vi "wd_append (Time).vi"(6 "data type":T7, 7 "data":timestamp[](array[timestamp]), 8 "error in (no error)":errorcluster, 9 "channel index":u32, 11 "meta in":T1={"TargetFile"=path "", "StreamMode"=enum."File", "Append?"=FALSE, "ChunkSize"=0, "TimeColumnMode"=enum."Empty", "TimestampFormat"="", "AbsoluteTime?"=FALSE, "FileAttribute "={"Creator"="", "Title"="", "SheetName"=""}, "Column"=[], "FileRef"=refnum, "MemoryRef"=[], "RecordInfo"=[], " ChannelPreviousInfo"=[], "ChannelFirstRecord"=[], "PredefinedFormattedValueLength"=20, "DiskTemplate"={"XMLRef"=[refnum, refnum, refnum, refnum, refnum, refnum], "ZipPath"=path "", "MetaFile"={"Ref"=refnum, "NextRow"=0, "NextPosition"=0, "Block"=[]}, "TempFolder"=path ""}}) -> (0 "error out":errorcluster, 3 "meta out":T1={"TargetFile"=path "", "StreamMode"=enum."File", "Append?"=FALSE, "ChunkSize"=0, "TimeColumnMode"=enum."Empty", "TimestampFormat"="", "AbsoluteTime?"=FALSE, "FileAttribute "={"Creator"="", "Title"="", "SheetName"=""}, "Column"=[], "FileRef"=refnum, "MemoryRef"=[], "RecordInfo"=[], " ChannelPreviousInfo"=[], "ChannelFirstRecord"=[], "PredefinedFormattedValueLength"=20, "DiskTemplate"={"XMLRef"=[refnum, refnum, refnum, refnum, refnum, refnum], "ZipPath"=path "", "MetaFile"={"Ref"=refnum, "NextRow"=0, "NextPosition"=0, "Block"=[]}, "TempFolder"=path ""}})   [LabVIEW 2017, in "NI_ExcelFile.lvlib"]
uses:
  <vilib>/express/express shared/NI_ExcelFile/NI_ExcelFile.lvlib
  <vilib>/express/express shared/NI_ExcelFile/Ctrls/DataType.ctl
  <vilib>/express/express shared/NI_ExcelFile/Ctrls/MainData.ctl
  <vilib>/express/express shared/NI_ExcelFile/Ctrls/StreamMode.ctl
  <vilib>/express/express shared/NI_ExcelFile/Ctrls/TimeColumnMode.ctl
  <vilib>/express/express shared/NI_ExcelFile/Ctrls/FileAttribute.ctl
  <vilib>/express/express shared/NI_ExcelFile/Ctrls/Columns.ctl
  <vilib>/express/express shared/NI_ExcelFile/Ctrls/ColumnInfo.ctl
  <vilib>/express/express shared/NI_ExcelFile/Ctrls/wd_recordInfo.ctl
  <vilib>/express/express shared/NI_ExcelFile/Ctrls/disk_TemplateFile.ctl
  <vilib>/express/express shared/NI_ExcelFile/Ctrls/meta_file.ctl
  <vilib>/express/express shared/NI_ExcelFile/Ctrls/meta_Block.ctl
  <vilib>/express/express shared/NI_ExcelFile/Ctrls/meta_BlockType.ctl
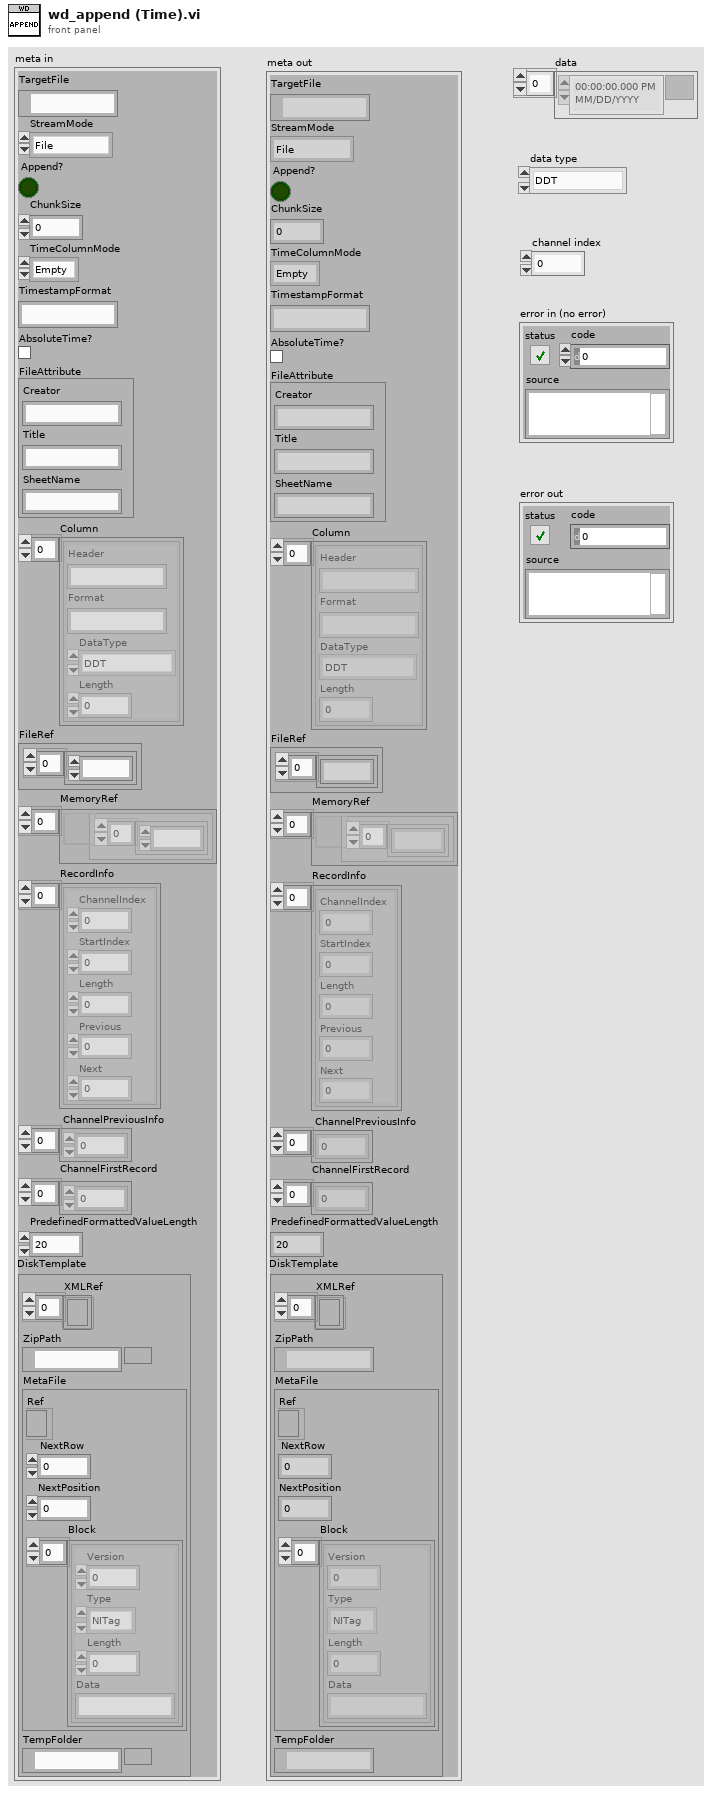
[diagram p1: front panel]
types:
  T1 = typedef "NI_ExcelFile.lvlib/MainData.ctl" = cluster{"TargetFile":path, "StreamMode":T2, "Append?":bool, "ChunkSize":u64, "TimeColumnMode":T3, "TimestampFormat":string, "AbsoluteTime?":bool, "FileAttribute ":T4, "Column":T5, "FileRef":refnum<k1>, "MemoryRef":refnum<data-value>[], "RecordInfo":T8[], " ChannelPreviousInfo":u32[], "ChannelFirstRecord":u32[], "PredefinedFormattedValueLength":i64, "DiskTemplate":T9}
  T2 = typedef "NI_ExcelFile.lvlib/StreamMode.ctl" = enum16{"File", "Memory"}
  T3 = typedef "NI_ExcelFile.lvlib/TimeColumnMode.ctl" = enum16{"Empty", "OnePerCh", "One"}
  T4 = typedef "NI_ExcelFile.lvlib/FileAttribute.ctl" = cluster{"Creator":string, "Title":string, "SheetName":string}
  T5 = typedef "NI_ExcelFile.lvlib/Columns.ctl" = T6[]
  T6 = typedef "NI_ExcelFile.lvlib/ColumnInfo.ctl" = cluster{"Header":string, "Format":string, "DataType":T7, "Length":u64}
  T7 = typedef "NI_ExcelFile.lvlib/DataType.ctl" = enum16{"DDT", "WFM", "Array of STR", "Array of DBL", "Array of I8", "Array of I16", "Array of I32", "Array of I64", "Array of SGL", "Array of U8", "Array of U16", "Array of U32", "Array of U64", "Array of Time"}
  T8 = typedef "NI_ExcelFile.lvlib/wd_recordInfo.ctl" = cluster{"ChannelIndex":u32, "StartIndex":u64, "Length":u64, "Previous":i32, "Next":i32}
  T9 = typedef "NI_ExcelFile.lvlib/disk_TemplateFile.ctl" = cluster{"XMLRef":refnum<file>[], "ZipPath":path, "MetaFile":T10, "TempFolder":path}
  T10 = typedef "NI_ExcelFile.lvlib/meta_file.ctl" = cluster{"Ref":refnum<file>, "NextRow":i32, "NextPosition":i64, "Block":T11[]}
  T11 = typedef "NI_ExcelFile.lvlib/meta_Block.ctl" = cluster{"Version":u16, "Type":T12, "Length":i32, "Data":string}
  T12 = typedef "NI_ExcelFile.lvlib/meta_BlockType.ctl" = enum16{"NITag", "File", "Column"}
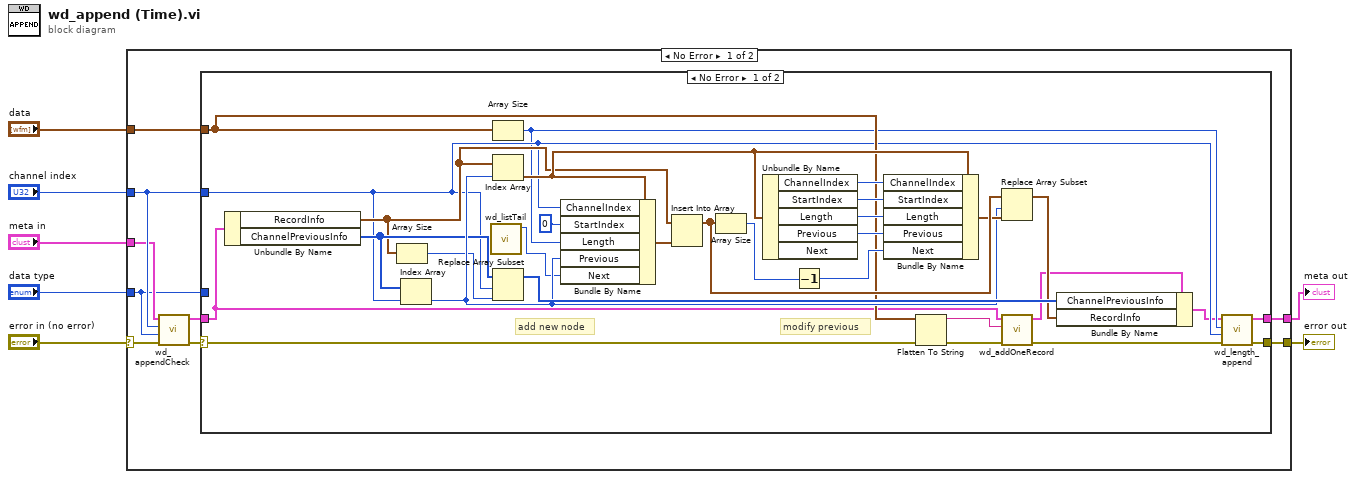
[diagram p0: block diagram]
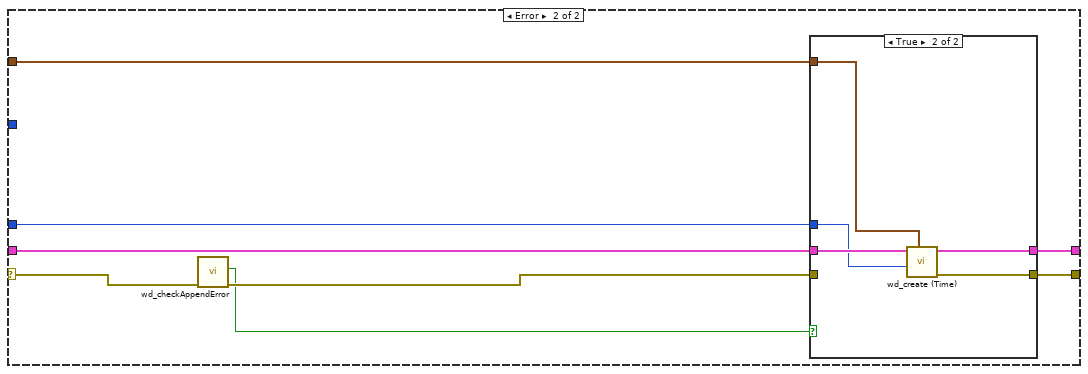
[diagram p2: hidden frame]
diagram:
  n1 = case shown="No Error" "error in (no error)" {
    selector: "error in (no error)" -> [w8 w63]
    tunnel: "data type" -> [w10 _]
    tunnel: "channel index" -> [w13 _]
    tunnel: "meta in" -> [w12 w62]
    tunnel: [w16 w62] -> w4
    tunnel: [w15 w63] -> w3
    tunnel: "data" -> [w14 _]
    frame No Error {
      n2 = call <vilib>:"wd_appendCheck.vi"("error in (no error)"=w8, "DataType"=w10, "channel index (0)"=w13, "data in"=w12) -> ("error out"=w9:errorcluster, "data out"=w11:T1)  [unwired: 6 in]
      n3 = case shown="No Error" w9 {
        selector: w9 -> [w20 w49]
        tunnel: [w18 w50] -> w15
        tunnel: w11 -> [w24 w52]
        tunnel: w14 -> [w29 w54]
        tunnel: [w21 w51] -> w16
        tunnel: w13 -> [w26 _]
        tunnel: w10 -> [_ w53]
        frame No Error {
          # "modify previous"
          # "add new node"
          n4 = Unbundle By Name(w24) -> ("RecordInfo"=w30:T8[], "ChannelPreviousInfo"=w31:u32[])
          n5 = Array Size(array=w30) -> (size(s)=w32:i32)
          n6 = Index Array(array=w31, index=w26) -> (element=w34:u32)
          n7 = call <vilib>:"wd_listTail.vi"() -> ("list tail"=w17:i32)  [unwired: 11 in]
          n8 = Array Size(array=w29) -> (size(s)=w25:i32)
          n9 = Index Array(array=w30, index=w34) -> (element=w43:T8)
          n10 = Replace Array Subset(array=w31, new element=w32, index=w26) -> (w46:u32[])
          n11 = Bundle By Name(cluster=w43, "ChannelIndex"=w26, "StartIndex"=u64 0 ("Start Index"), "Length"=w25, "Previous"=w34, "Next"=w17) -> (w44:T8)
          n12 = Insert Into Array(array=w30, new element=w44) -> (w36:T8[])  [unwired: 1 in]
          n13 = Array Size(array=w36) -> (size(s)=w38:i32)
          n14 = Unbundle By Name(w43) -> ("ChannelIndex"=w42:u32, "StartIndex"=w41:u64, "Length"=w40:u64, "Previous"=w39:i32)  [unwired: 1 out]
          n15 = Decrement(x=w38) -> (x-1=w37:i32)
          n16 = Bundle By Name(cluster=w43, "ChannelIndex"=w42, "StartIndex"=w41, "Length"=w40, "Previous"=w39, "Next"=w37) -> (w35:T8)
          n17 = Flatten To String(anything=w29, error in (no error)=w20) -> (data string=w28:string, error out=w27:errorcluster)  [unwired: 2 in, 1 out]
          n18 = Replace Array Subset(array=w36, new element=w35, index=w34) -> (w33:T8[])
          n19 = call <vilib>:"wd_addOneRecord.vi"("error in (no error)"=w27, "data"=w28, "meta in"=w24) -> ("error out"=w19:errorcluster, "meta out"=w23:T1)  [unwired: 7 in]
          n20 = Bundle By Name(cluster=w23, "ChannelPreviousInfo"=w46, "RecordInfo"=w33) -> (w22:T1)
          n21 = call <vilib>:"wd_length_append.vi"("error in (no error)"=w19, "channel index (0)"=w26, "data size"=w25, "meta in"=w22) -> ("error out"=w18:errorcluster, "meta out"=w21:T1)  [unwired: 6 in]
        }
        frame Error {
          n22 = call <vilib>:"wd_checkAppendError.vi"("error in (no error)"=w49) -> ("error out"=w48:errorcluster, "special error?"=w47:bool)  [unwired: 9 in]
          n23 = case shown="True" w47 {
            tunnel: w52 -> [w56 w61]
            tunnel: w54 -> [_ w57]
            tunnel: w53 -> [_ w60]
            tunnel: w48 -> [w55 _]
            tunnel: [w56 w59] -> w51
            tunnel: [w55 w58] -> w50
            frame False {
            }
            frame True {
              n24 = call <vilib>:"wd_create (Time).vi"("data"=w57, "data type"=w60, "meta in"=w61) -> ("error out"=w58:errorcluster, "meta out"=w59:T1)  [unwired: 7 in]
            }
          }
        }
      }
    }
    frame Error {
    }
  }
  "meta out" <- w4
  "error out" <- w3
